vi "OLD_get_max_peaks.vi"(6 "Amplitudes":dbl[](array[numeric]), 7 "n->p indexes":i32[](array[numeric]), 9 "p->n indexes":i32[](array[numeric]), 10 "Locations":dbl[](array[numeric]), 11 "peak times":dbl[](array[numeric])) -> (3 "Correted Peaks":cluster{"Array":dbl[], "Array":dbl[]})   [LabVIEW 2020]
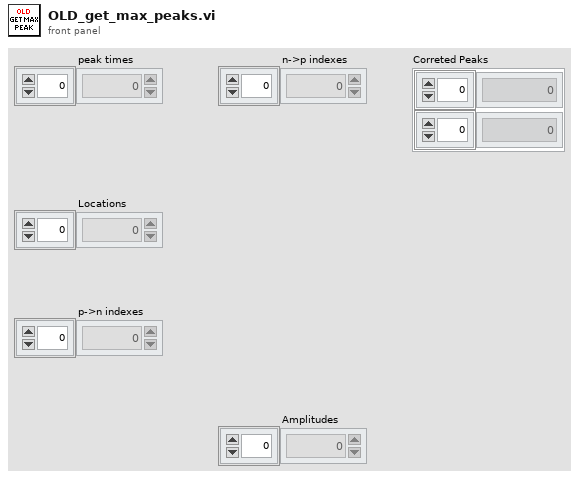
[diagram p1: front panel]
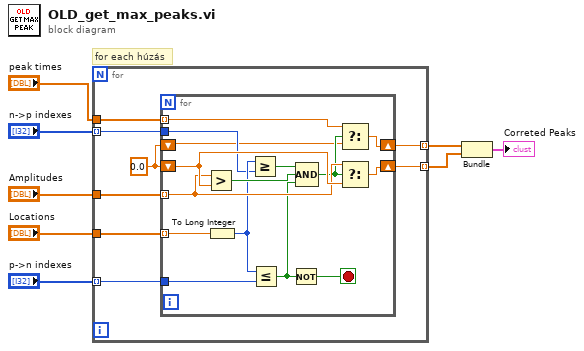
[diagram p0: block diagram]
diagram:
  # "for each húzás"
  n1 = for {
    tunnel: "Locations" -> [w16]
    tunnel: "Amplitudes" -> [w14]
    tunnel: [w15] -> w7 mode=indexing
    tunnel: "n->p indexes" -> [w13] mode=indexing
    tunnel: "p->n indexes" -> [w12] mode=indexing
    tunnel: [w11] -> w6 mode=indexing
    tunnel: "peak times" -> [w10]
    w9 = 0.0
    n2 = for {
      tunnel: w13 -> [w25]
      tunnel: w12 -> [w24]
      tunnel: w16 -> [w17] mode=indexing
      shift-right: [w31] -> w15
      shift-left: w9 -> [w30]
      tunnel: w14 -> [w29] mode=indexing
      shift-right: [w23] -> w11
      shift-left: w9 -> [w21]
      tunnel: w10 -> [w20] mode=indexing
      stop <- w19 stop-if-true
      n3 = Greater?(x=w29, y=w30) -> (0:w28:bool)
      n4 = To Long Integer(number=w17) -> (32bit integer=w26:i32)
      n5 = Greater Or Equal?(x=w26, y=w25) -> (x >= y?=w27:bool)
      n6 = Less Or Equal?(x=w26, y=w24) -> (x <= y?=w18:bool)
      n7 = Not(x=w18) -> (.not. x?=w19:bool)
      n8 = Compound Arithmetic op=AND(w27, w28, w18) -> (w22:bool)
      n9 = Select(t=w20, s=w22, f=w21) -> (s? t:f=w23:dbl)
      n10 = Select(t=w29, s=w22, f=w30) -> (s? t:f=w31:dbl)
    }
  }
  n11 = Bundle(w6, w7) -> (→"Correted Peaks":cluster{dbl[], dbl[]})  [unwired: 1 in]
